vi "Update.vi"(7 "Row":i32, 8 "error in (no error)":errorcluster, 9 "Workspace":T1, 10 "Routine":T2=enum."Dispense on Plate", 11 "Assembly Run in":refnum<class "Assembly Run.lvclass">) -> (0 "error out":errorcluster, 3 "Assembly Run out":refnum<class "Assembly Run.lvclass">)   [LabVIEW 2016, in "Assembly Run.lvclass"]
uses:
  Assembly Run.lvclass
  Routine/Routine Enum.ctl
  Routine/Routine.lvclass
  Workspace/Fixture Enum.ctl
  Workspace/Fixture.lvclass
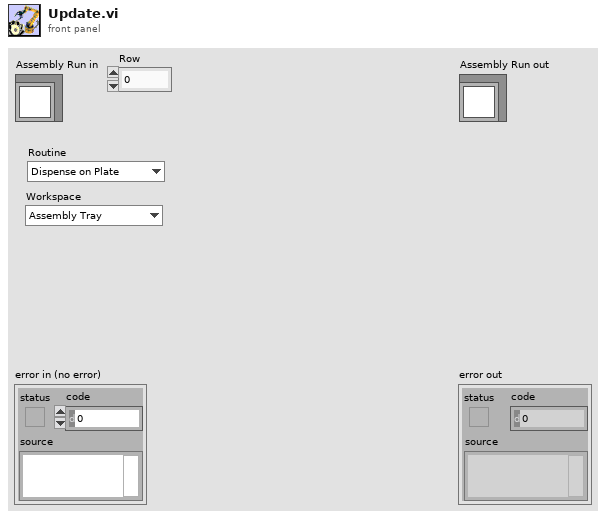
[diagram p1: front panel]
types:
  T1 = typedef "Fixture.lvclass/Fixture Enum.ctl" = enum16{"Assembly Tray", "Syringe Space", "Component", "Pick Up Tool", "Current Position"}
  T2 = typedef "Routine.lvclass/Routine Enum.ctl" = enum16{"Primary Pick Up", "Pick Up All", "Put Down Secondary", "Put Down All", "Release Syringe", "Secondary Pick Up", "Secure Syringe", "Dispense on Plate", "Dispense on Kapton", "Dispense on Sensor"}
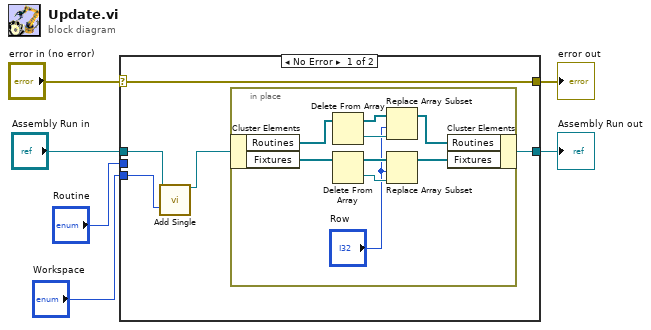
[diagram p0: block diagram]
diagram:
  n1 = case shown="No Error" "error in (no error)" {
    selector: "error in (no error)" -> [w11 w22]
    tunnel: [w11 w22] -> w5
    tunnel: [w10 w21] -> w3
    tunnel: "Assembly Run in" -> [w8 w21]
    tunnel: "Routine" -> [_ _]
    tunnel: "Workspace" -> [w9 _]
    frame No Error {
      n2 = call-dynamic "Add Single.vi"("UI in"=w8, "Fixture"=w9) -> ("UI out"=w7:refnum<class "Assembly Run.lvclass">)  [unwired: 16 in, 1 out]
      n3 = in-place {
        n4 = in-place-cluster #1(w7) -> ("Routines"=w16:refnum<class "Routine.lvclass">[], "Fixtures"=w15:refnum<class "Fixture.lvclass">[])
        n5 = Delete From Array(array=w16) -> (deleted portion=w18:refnum<class "Routine.lvclass">, array with subset deleted=w17:refnum<class "Routine.lvclass">[])  [unwired: 2 in]
        n6 = Delete From Array(array=w15) -> (deleted portion=w19:refnum<class "Fixture.lvclass">, array with subset deleted=w20:refnum<class "Fixture.lvclass">[])  [unwired: 2 in]
        n7 = Replace Array Subset(array=w17, new element=w18, index="Row") -> (w14:refnum<class "Routine.lvclass">[])
        n8 = Replace Array Subset(array=w20, new element=w19, index="Row") -> (w13:refnum<class "Fixture.lvclass">[])
        n9 = in-place-cluster #1("Routines"=w14, "Fixtures"=w13) -> (w10:refnum<class "Assembly Run.lvclass">)
      }
    }
    frame Error {
    }
  }
  "error out" <- w5
  "Assembly Run out" <- w3
